vi "Write DC Pins.vi"(8 "error in (no error)":errorcluster, 10 "DC Pins":string[](array[string]), 11 "Harmonics in":refnum<class "Harmonics.lvclass">) -> (0 "error out":errorcluster, 3 "Harmonics out":refnum<class "Harmonics.lvclass">)   [LabVIEW 2016, in "Harmonics.lvlib" / "Harmonics.lvclass"]
uses:
  Harmonics.lvclass
  Harmonics.lvclass/Harmonics.ctl
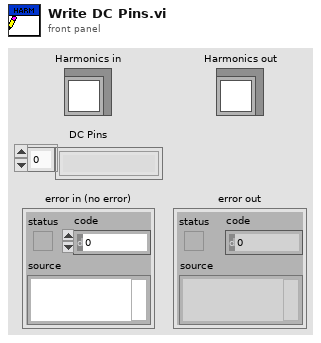
[diagram p1: front panel]
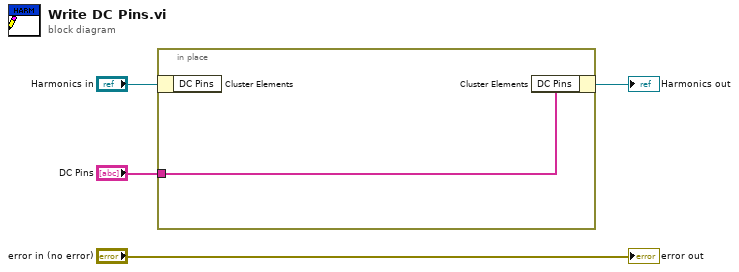
[diagram p0: block diagram]
diagram:
  n1 = in-place {
    in-place-border: "DC Pins" -> [w5]
    n2 = in-place-cluster #1("Harmonics in") -> ()  [unwired: 1 out]
    n3 = in-place-cluster #1("DC Pins"=w5) -> (→"Harmonics out":refnum<class "Harmonics.lvclass">)
  }
  "error out" <- "error in (no error)"
